vi "Exponent Function.vi"(9 "Exponent":dbl, 10 "Left In":dbl, 11 "Right In":dbl) -> (2 "Right Out":dbl, 3 "Left Out":dbl)   [LabVIEW 2012]
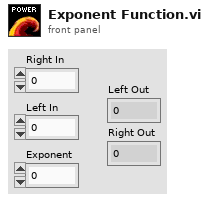
[diagram p1: front panel]
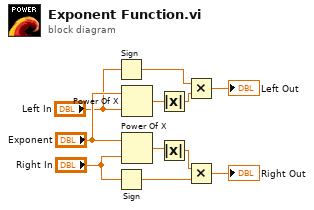
[diagram p0: block diagram]
diagram:
  n1 = Sign(1:"Left In") -> (0:w6:dbl)
  n2 = Sign(1:"Right In") -> (0:w3:dbl)
  n3 = Power Of X(1:"Left In", 2:"Exponent") -> (0:w7:dbl)
  n4 = Power Of X(1:"Right In", 2:"Exponent") -> (0:w8:dbl)
  n5 = Absolute Value(x=w7) -> (abs(x)=w5:dbl)
  n6 = Absolute Value(x=w8) -> (abs(x)=w4:dbl)
  n7 = Multiply(x=w6, y=w5) -> (x*y=→"Left Out":dbl)
  n8 = Multiply(x=w4, y=w3) -> (x*y=→"Right Out":dbl)
